vi "Graphics-Show Y-Autoscale Context Menu.vi"(1 "Y-autoscale":enum16{"Off", "Min", "Max", "All"}(ring), 2 "Menu in":refnum<k9>) -> ()   [LabVIEW 2020]
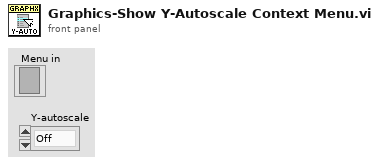
[diagram p1: front panel]
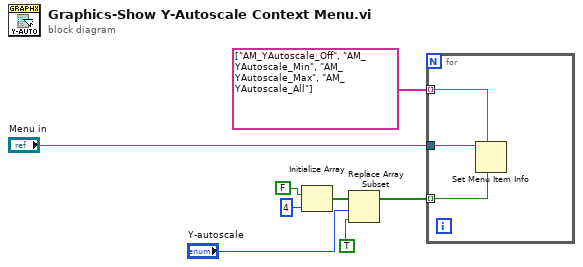
[diagram p0: block diagram]
diagram:
  n1 = Initialize Array(FALSE, 4 ("dimension size")) -> (w4:bool[])
  n2 = Replace Array Subset(array=w4, new element=TRUE ("new element/subarray"), index="Y-autoscale") -> (w7:bool[])
  n3 = for {
    tunnel: "Menu in" -> [w11]
    tunnel: w7 -> [w10] mode=indexing
    tunnel: string[] ["AM_YAutoscale_Off", "AM_YAutoscale_Min", "AM_YAutoscale_Max", "AM_YAutoscale_All"] -> [w9] mode=indexing
    n4 = Set Menu Item Info(6:w10, 7:w9, 11:w11) -> ()  [unwired: 4 in, 2 out]
  }
